vi "MergePropertyNode.vi"   [LabVIEW 2016]
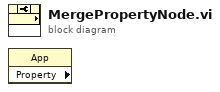
[diagram p0: block diagram]
diagram:
  n1 = property class="App" props=[]() -> ()  [unwired: 2 in, 3 out]
